vi "GetNumericFloatFromReference.vi"(10 "error in (no error)":errorcluster, 11 "reference":refnum<vi>) -> (2 "error out":errorcluster, 3 "Value":dbl)   [LabVIEW 2019, in "Utilities.lvlib"]
uses:
  Utilities.lvlib
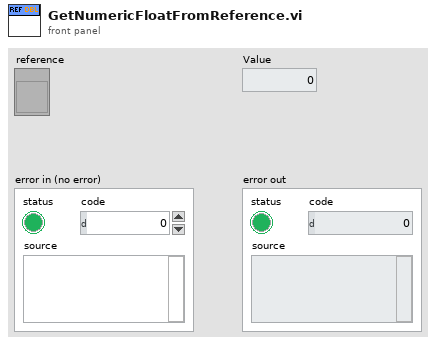
[diagram p1: front panel]
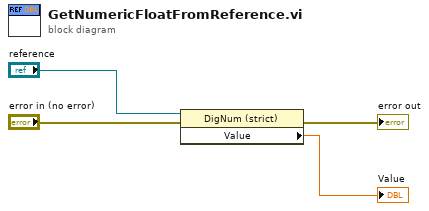
[diagram p0: block diagram]
diagram:
  n1 = property class="DigNum (strict)"(reference="reference", error in="error in (no error)") -> (error out=→"error out":errorcluster, "Value"=→"Value":dbl)  [unwired: 1 out]
